vi "Week_4_4.1_Example-2.vi"() -> ()   [LabVIEW 2015]
panel:
  out "Waveform Graph":dynamicdata(graph)
  out "RMS":dbl format="%#_13g"
  out "Positive Peak":dbl format="%#_13g"
  out "Peak To Peak":dbl format="%#_13g"
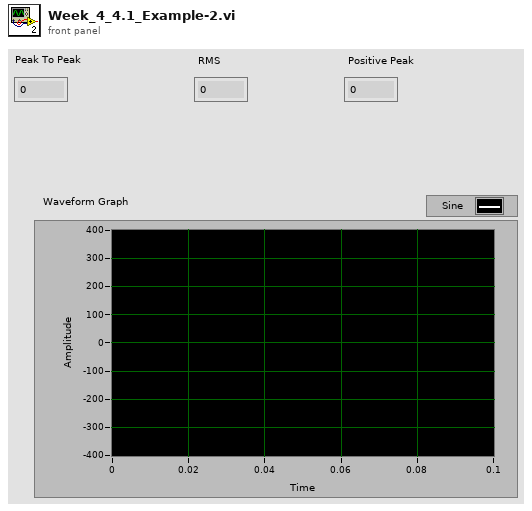
[diagram p1: front panel]
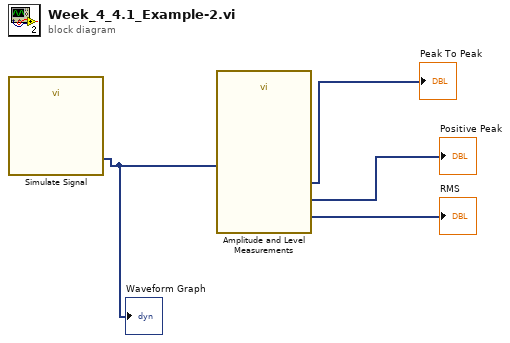
[diagram p0: block diagram]
diagram:
  n1 = call "Simulate Signal"() -> ("Sine"=w1:dynamicdata)  [unwired: 14 in, 1 out]
  "Waveform Graph" <- w1
  n2 = call "Amplitude and Level Measurements"("Signals"=w1) -> ("RMS"=→"RMS":dynamicdata, "Positive Peak"=→"Positive Peak":dynamicdata, "Peak to Peak"=→"Peak To Peak":dynamicdata)  [unwired: 11 in, 1 out]
